vi "Const Frame Empty Data.vi"(11 "frame number":string) -> (3 "frame data":T1)   [LabVIEW 2018, in "Main Panel.lvlib" / "Main Panel.lvclass"]
uses:
  Main Panel.lvclass
  Frame Analizer/frame data.ctl
  Frame Analizer/frame title.ctl
  Frame Analizer/frame basic data.ctl
  Frame Analizer/frame o data.ctl
  Frame Analizer/frame bp data.ctl
  Frame Analizer/frame c data.ctl
  Frame Analizer/frame w data.ctl
  Frame Analizer/frame i data.ctl
  Frame Analizer/frame b data.ctl
  Frame Analizer/Data Parser.lvclass
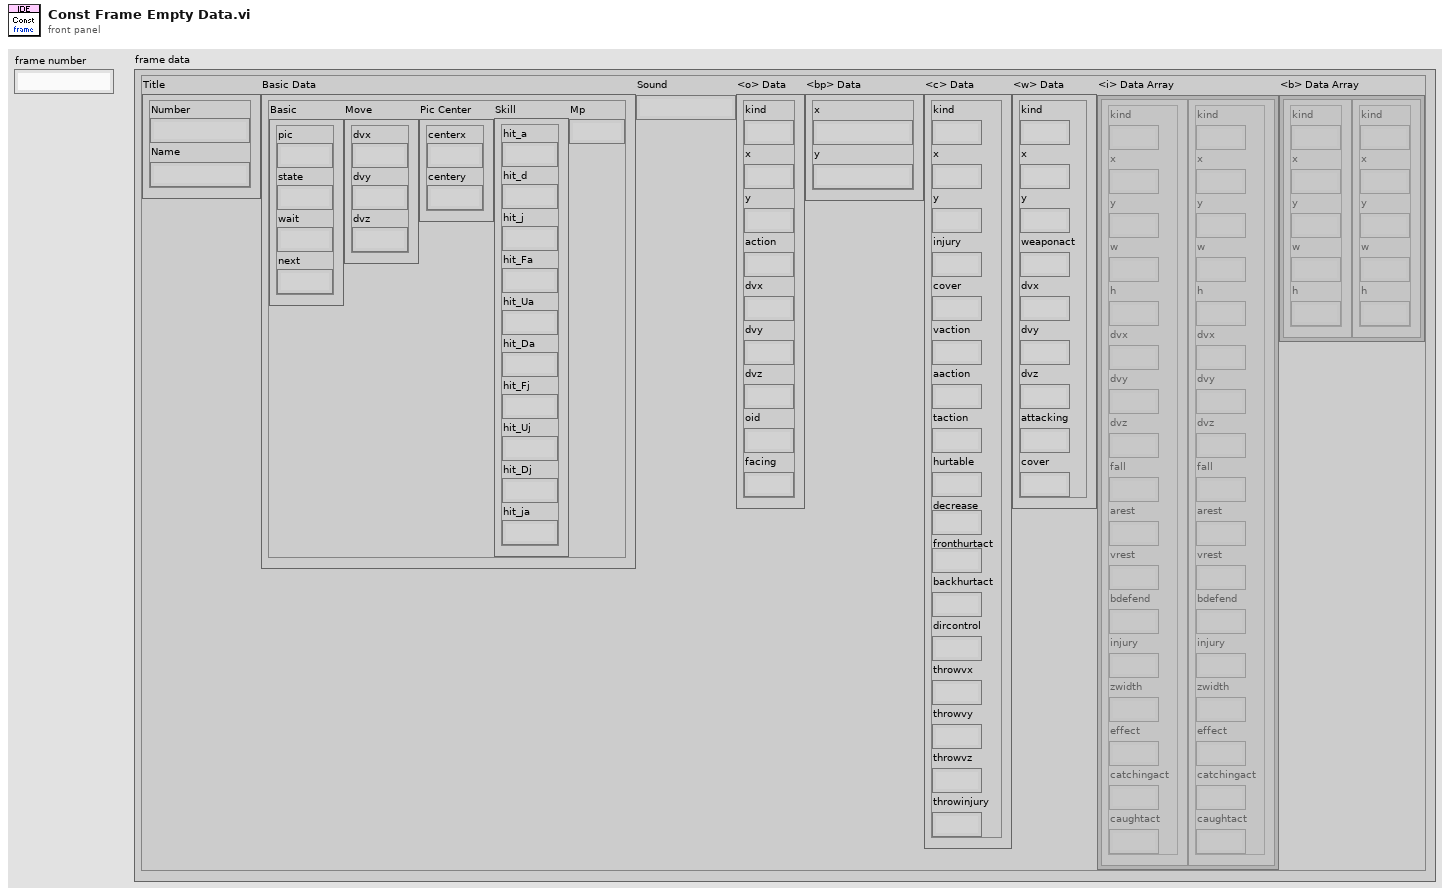
[diagram p1: front panel]
types:
  T1 = typedef "Data Parser.lvclass/frame data.ctl" = cluster{"Title":T2, "Basic Data":T3, "Sound":string, "<o> Data":T4, "<bp> Data":T5, "<c> Data":T6, "<w> Data":T7, "<i> Data Array":T8[], "<b> Data Array":T9[]}
  T2 = typedef "Data Parser.lvclass/frame title.ctl" = cluster{"Number":string, "Name":string}
  T3 = typedef "Data Parser.lvclass/frame basic data.ctl" = cluster{"Basic":cluster{"pic":string, "state":string, "wait":string, "next":string}, "Move":cluster{"dvx":string, "dvy":string, "dvz":string}, "Pic Center":cluster{"centerx":string, "centery":string}, "Skill":cluster{"hit_a":string, "hit_d":string, "hit_j":string, "hit_Fa":string, "hit_Ua":string, "hit_Da":string, "hit_Fj":string, "hit_Uj":string, "hit_Dj":string, "hit_ja":string}, "Mp":string}
  T4 = typedef "Data Parser.lvclass/frame o data.ctl" = cluster{"kind":string, "x":string, "y":string, "action":string, "dvx":string, "dvy":string, "dvz":string, "oid":string, "facing":string}
  T5 = typedef "Data Parser.lvclass/frame bp data.ctl" = cluster{"x":string, "y":string}
  T6 = typedef "Data Parser.lvclass/frame c data.ctl" = cluster{"kind":string, "x":string, "y":string, "injury":string, "cover":string, "vaction":string, "aaction":string, "taction":string, "hurtable":string, "decrease":string, "fronthurtact":string, "backhurtact":string, "dircontrol":string, "throwvx":string, "throwvy":string, "throwvz":string, "throwinjury":string}
  T7 = typedef "Data Parser.lvclass/frame w data.ctl" = cluster{"kind":string, "x":string, "y":string, "weaponact":string, "dvx":string, "dvy":string, "dvz":string, "attacking":string, "cover":string}
  T8 = typedef "Data Parser.lvclass/frame i data.ctl" = cluster{"kind":string, "x":string, "y":string, "w":string, "h":string, "dvx":string, "dvy":string, "dvz":string, "fall":string, "arest":string, "vrest":string, "bdefend":string, "injury":string, "zwidth":string, "effect":string, "catchingact":string, "caughtact":string}
  T9 = typedef "Data Parser.lvclass/frame b data.ctl" = cluster{"kind":string, "x":string, "y":string, "w":string, "h":string}
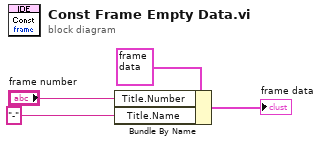
[diagram p0: block diagram]
diagram:
  n1 = Bundle By Name(cluster=T1 {"Title"={"Number"="", "Name"=""}, "Basic Data"={"Basic"={"pic"="", "state"="", "wait"="", "next"=""}, "Move"={"dvx"="", "dvy"="", "dvz"=""}, "Pic Center"={"centerx"="", "centery"=""}, "Skill"={"hit_a"="", "hit_d"="", "hit_j"="", "hit_Fa"="", "hit_Ua"="", "hit_Da"="", "hit_Fj"="", "hit_Uj"="", "hit_Dj"="", "hit_ja"=""}, "Mp"=""}, "Sound"="", "<o> Data"={"kind"="", "x"="", "y"="", "action"="", "dvx"="", "dvy"="", "dvz"="", "oid"="", "facing"=""}, "<bp> Data"={"x"="", "y"=""}, "<c> Data"={"kind"="", "x"="", "y"="", "injury"="", "cover"="", "vaction"="", "aaction"="", "taction"="", "hurtable"="", "decrease"="", "fronthurtact"="", "backhurtact"="", "dircontrol"="", "throwvx"="", "throwvy"="", "throwvz"="", "throwinjury"=""}, "<w> Data"={"kind"="", "x"="", "y"="", "weaponact"="", "dvx"="", "dvy"="", "dvz"="", "attacking"="", "cover"=""}, "<i> Data Array"=[], "<b> Data Array"=[]} ("Data.frame data"), "Title.Number"="frame number", "Title.Name"="-" ("title.name")) -> (→"frame data":T1)
